vi "Write Data.vi"(8 "error in (no error)":errorcluster, 9 "Publication Time":timestamp, 10 "Value":variant, 11 "ActorMessage in":refnum<class "ActorMessage.lvclass">) -> (0 "error out":errorcluster, 3 "ActorMessage out":refnum<class "ActorMessage.lvclass">)   [LabVIEW 2015, in "Mediator.lvlib" / "ActorMessage.lvclass"]
doc: "<License>\nCopyright © 2017 Composed Systems, LLC | All rights reserved\nwww.composed.io\n\nAuthor: Ethan Stern <ethan.stern@composed.io>\n\nThis software is provided \"AS IS\" WITHOUT WARRANTIES, either express or implied, AND IS FOR EDUCATIONAL PURPOSES ONLY.\n</License>"
uses:
  ActorMessage.lvclass
  ActorMessage.lvclass/ActorMessage.ctl
  Transport Messages/Notification Msg/Notification Msg.lvclass
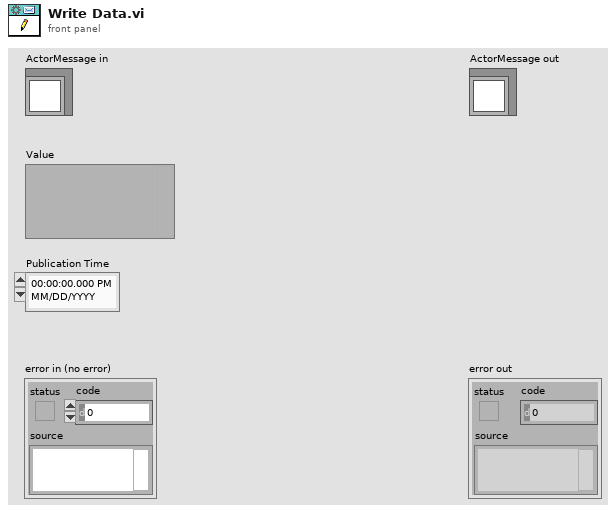
[diagram p1: front panel]
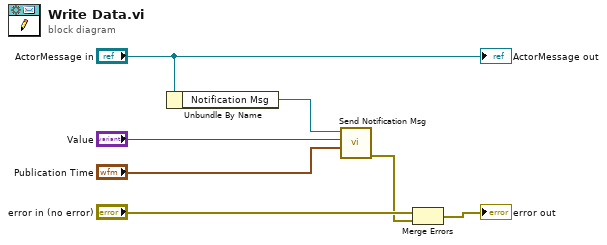
[diagram p0: block diagram]
diagram:
  n1 = Unbundle By Name("ActorMessage in") -> ("Notification Msg"=w6:refnum<class "Notification Msg.lvclass">)
  n2 = call "Send Notification Msg.vi"("Publication Time (Use Current Time)"="Publication Time", "Value"="Value", "Notification Msg in"=w6) -> ("error out"=w1:errorcluster)  [unwired: 8 in]
  n3 = Merge Errors("error in (no error)", w1) -> (→"error out":errorcluster)
  "ActorMessage out" <- "ActorMessage in"
